vi "beginABCPassPlay.vi"(8 "error in (no error)":errorcluster, 10 "Game in":refnum<class "Game.lvclass">, 11 "ABCPassPlay in":refnum<class "ABCPassPlay.lvclass">) -> (0 "error out":errorcluster, 2 "result":bool, 3 "ABCPassPlay out":refnum<class "ABCPassPlay.lvclass">)   [LabVIEW 2020, in "ABCPassPlay.lvclass"]
uses:
  ABCPassPlay.lvclass
  Game_class/Game.lvclass
  Referee_class/command_interpreted.ctl
  Team_class/OffensivePlay.ctl
  Game_class/Game.lvclass/Game.ctl
  Referee_class/Referee.lvclass/Referee.ctl
  Team_class/Team.lvclass/Team.ctl
  Game_class/Read OffensiveTeam.vi
  Team_class/Read RobotRef.vi
  Team_class/Read OffensivePlay.vi
  Game_class/Read Referee.vi
  Game_class/Read Utilities.lvclass.vi
  Referee_class/Read command_interpreted.vi
  Ally_class/Ally.lvclass
  C:/Users/anton/Desktop/RoboIME/IC/SSL_AI/Team_class/Team.lvclass
  Referee_class/Referee.lvclass
  Utilities_class/Utilities.lvclass
  Robot_class/Robot.lvclass
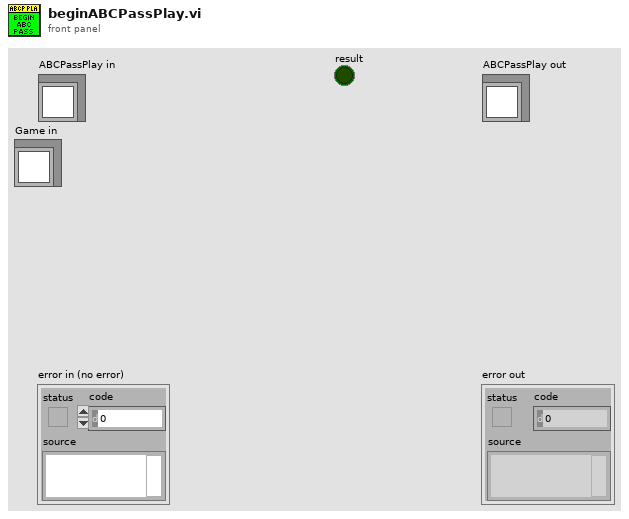
[diagram p1: front panel]
types:
  T1 = typedef "command_interpreted.ctl" = enum16{"Goal Ally", "Goal Enemy", "Ball Placement Enemy", "Ball Placement Ally", "Normal Half Time", "Extra Time  Break", "Extra Half Time", "None", "Post Game", "PKA Normal Start", "Prepare Kickoff Ally", "PKE Normal Start", "Prepare Kickoff Enemy", "Force Start", "Halt", "Timeout", "Prepare Penalty Ally", "Prepare Penalty Enemy", "PPA NormalStart", "PPE Normal Start", "Indirect Free Ally", "Direct Free Enemy", "Direct Free Ally", "Indirect Free Enemy", "Stop"}
  T2 = typedef "OffensivePlay.ctl" = enum16{"5RobotsPassGamePlay", "5PreparePassGame", "5RobotsKeeperGame", "KeeperPassToStriker", "5RobotsNormalGamePlay", "PrepareKeeperPass", "ACBPass", "ABCPass", "PrepareTriplePass", "TableWithStriker", "TableWith2ndStrikerPlay", "PrepareDoublePass", "PrepareRollToPass", "SimplePass", "PreparePass", "PassToStriker", "BallOutOfField", "PassTo2ndStriker", "StopOffensive", "Prepare Penalty Enemy", "EnemyPossessionAtEnemyField", "EnemyPossesionAtOurField", "TestPlay", "PreparePenaltyAlly", "KickPenaltyAlly", "PrepareKickoffAlly", "PrepareKickoffEnemy", "IndirectEnemy", "DirectEnemy", "PreparePassInGame1", "NormalGame", "DirectKick", "Pass", "Halt", "Timeout", "PassPlay", "PenaltyEnemy"}
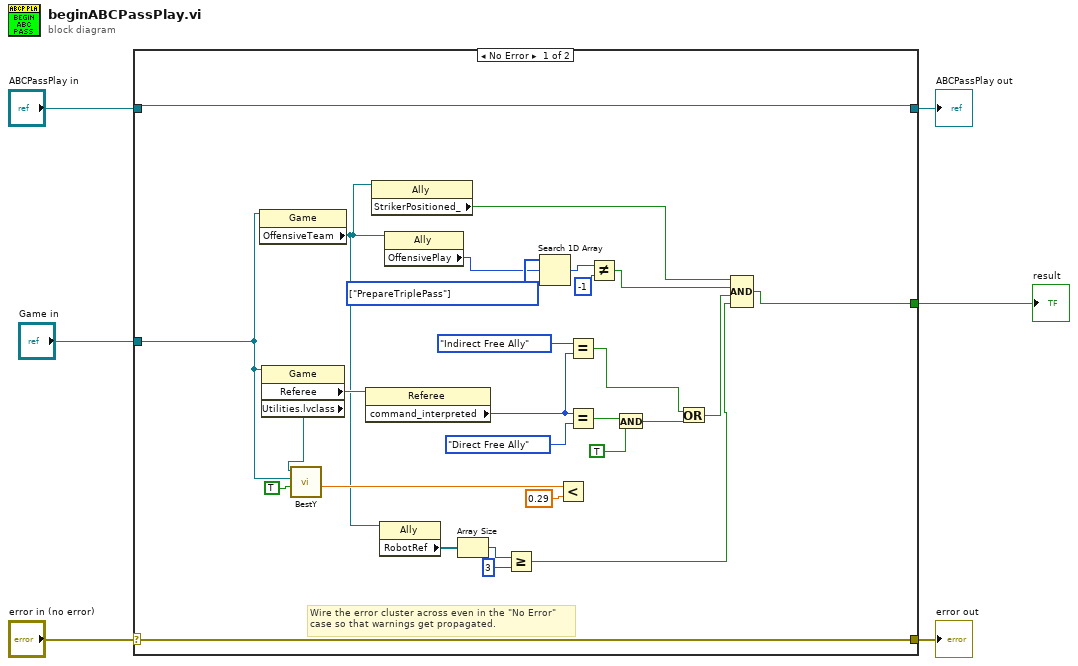
[diagram p0: block diagram]
diagram:
  n1 = case shown="No Error" "error in (no error)" {
    selector: "error in (no error)" -> [w33 w36]
    tunnel: [w33 w36] -> w5
    tunnel: [w34 w35] -> w3
    tunnel: "ABCPassPlay in" -> [w34 w35]
    tunnel: "Game in" -> [w14 _]
    tunnel: [w13 _] -> w1
    frame No Error {
      w10 = T2[] [enum."PrepareTriplePass"] items=["5RobotsPassGamePlay", "5PreparePassGame", "5RobotsKeeperGame", "KeeperPassToStriker", "5RobotsNormalGamePlay", "PrepareKeeperPass", "ACBPass", "ABCPass", "PrepareTriplePass", "TableWithStriker", "TableWith2ndStrikerPlay", "PrepareDoublePass", "PrepareRollToPass", "SimplePass", "PreparePass", "PassToStriker", "BallOutOfField", "PassTo2ndStriker", "StopOffensive", "Prepare Penalty Enemy", "EnemyPossessionAtEnemyField", "EnemyPossesionAtOurField", "TestPlay", "PreparePenaltyAlly", "KickPenaltyAlly", "PrepareKickoffAlly", "PrepareKickoffEnemy", "IndirectEnemy", "DirectEnemy", "PreparePassInGame1", "NormalGame", "DirectKick", "Pass", "Halt", "Timeout", "PassPlay", "PenaltyEnemy"] ("Array")
      # "Wire the error cluster across even in the \"No Error\"\ncase so that warnings get propagated."
      n2 = property class="Game"(reference=w14) -> ("OffensiveTeam"=w16:refnum<class "Ally.lvclass">)  [unwired: 1 in, 2 out]
      n3 = property class="Game"(reference=w14) -> ("Referee"=w32:refnum<class "Referee.lvclass">, "Utilities.lvclass"=w20:refnum<class "Utilities.lvclass">)  [unwired: 1 in, 2 out]
      n4 = call "BestY.vi"("Utilities in"=w20, "Game"=w14, "inimigos"=TRUE) -> ("Gap kick"=w26:dbl)  [unwired: 2 in, 4 out]
      n5 = property class="Referee"(reference=w32) -> ("command_interpreted"=w30:T1)  [unwired: 1 in, 2 out]
      n6 = property class="Ally"(reference=w16) -> ("StrikerPositioned_"=w25:bool)  [unwired: 1 in, 2 out]
      n7 = property class="Ally"(reference=w16) -> ("RobotRef"=w19:refnum<class "Robot.lvclass">[])  [unwired: 1 in, 2 out]
      n8 = property class="Ally"(reference=w16) -> ("OffensivePlay"=w9:T2)  [unwired: 1 in, 2 out]
      n9 = Array Size(array=w19) -> (size(s)=w18:i32)
      n10 = Greater Or Equal?(x=w18, y=3) -> (x >= y?=w15:bool)
      n11 = Search 1D Array(1D array=w10, element=w9) -> (index of element=w12:i32)  [unwired: 1 in]
      n12 = Less?(x=w26, y=0.29 ("Gap kick")) -> ()  [unwired: 1 out]
      n13 = Equal?(x=command_interpreted."Indirect Free Ally" ("command_interpreted"), y=w30) -> (x = y?=w22:bool)
      n14 = Equal?(x=w30, y=command_interpreted."Direct Free Ally" ("command_interpreted")) -> (x = y?=w24:bool)
      n15 = Not Equal?(x=w12, y=-1) -> (x != y?=w8:bool)
      n16 = And(x=w24, y=TRUE) -> (x .and. y?=w23:bool)
      n17 = Or(x=w22, y=w23) -> (x .or. y?=w21:bool)
      n18 = Compound Arithmetic op=AND(w25, w8, w21, w15) -> (w13:bool)
    }
    frame Error {
    }
  }
  "error out" <- w5
  "ABCPassPlay out" <- w3
  "result" <- w1
